vi "Open 4 Talon.vi"   [LabVIEW 2017]
uses:
  <vilib>/Rock Robotics/WPI/ThirdParty/Phoenix-LabVIEW/Motor Controller/Controls/CTRE_Phoenix_MotorControl_NeutralMode.ctl
  <vilib>/Rock Robotics/WPI/RobotDrive/WPI_RobotDriveOpen2MotorWithExistingMotors.vi
types:
  T1 = typedef "CTRE_Phoenix_MotorControl_NeutralMode.ctl" = enum8{"EEPROMSetting", "Override to Coast", "Override to Brake"}
  T2 = typedef "WPI_MotorControlDeviceRef.ctl" = cluster{"DeviceStatus":errorcluster, "Type":T3, "PWM":cluster{"PWM Channel":T4, "DeadBand":T5}, "CAN":cluster{"Device Number":u8, "SetOutput VI Ref":variant, "GetOutput VI Ref":variant, "Enable VI Ref":variant, "Disable VI Ref":variant, "Data":variant}, "Invert":bool, "DIO PWM":cluster{"PWM \"Enable\" Channel":T4, "DIOChannel":T6, "PWM Rate":dbl}}
  T3 = typedef "WPI_MotorControlType.ctl" = enum16{"PWM", "CAN", "DIO PWM"}
  T4 = typedef "FPGA_DIOPWMChannel.ctl" = enum8{"PWM 0", "PWM 1", "PWM 2", "PWM 3", "PWM 4", "PWM 5", "PWM 6", "PWM 7", "PWM 8", "PWM 9", "PWM MXP 0", "PWM MXP 1", "PWM MXP 2", "PWM MXP 3", "PWM MXP 4", "PWM MXP 5", "PWM MXP 6", "PWM MXP 7", "PWM MXP 8", "PWM MXP 9", "Invalid"}
  T5 = typedef "WPI_PWMDeadband.ctl" = cluster{"Name":string, "maxPositivePwm":i32, "minPositivePwm":i32, "centerPwm":i32, "maxNegativePwm":i32, "minNegativePwm":i32, "angularRange":u16}
  T6 = typedef "FPGA_DIOChannel.ctl" = enum8{"DIO 0", "DIO 1", "DIO 2", "DIO 3", "DIO 4", "DIO 5", "DIO 6", "DIO 7", "DIO 8", "DIO 9", "DIO MXP 0", "DIO MXP 1", "DIO MXP 2", "DIO MXP 3", "DIO MXP 4", "DIO MXP 5", "DIO MXP 6", "DIO MXP 7", "DIO MXP 8", "DIO MXP 9", "DIO MXP 10", "DIO MXP 11", "DIO MXP 12", "DIO MXP 13", "DIO MXP 14", "DIO MXP 15", "SPI Port CS1", "SPI Port CS2", "SPI Port CS3", "SPI Port MISO", "SPI Port MOSI", "Invalid"}
  T7 = typedef "WPI_RobotDriveDevRef.ctl" = cluster{"DevStatus":errorcluster, "Motors[]":T2[], "Square Inputs":bool, "Max Output":dbl}
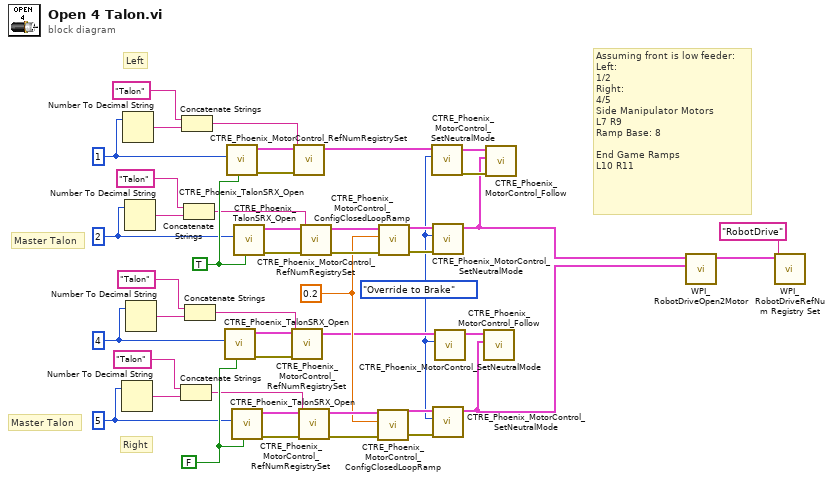
[diagram p0: block diagram]
diagram:
  w6 = CTRE_Phoenix_MotorControl_NeutralMode."Override to Brake" ("Motor Control Neutral Mode")
  w15 = 0.2 ("secondsFromNeutralToFull")
  w26 = FALSE ("Invert")
  w27 = TRUE ("Invert")
  w9 = u8 5 ("Device Number")
  w10 = u8 4 ("Device Number")
  w23 = u8 2 ("Device Number")
  w25 = u8 1 ("Device Number")
  # "Right"
  # "Left"
  # "Master Talon"
  # "Master Talon"
  # "Assuming front is low feeder:\nLeft:\n1/2\nRight:\n4/5\nSide Manipulator Motors\nL7 R9\nRamp Base: 8\n\nEnd Game Ramps\nL10 R11"
  n1 = Number To Decimal String(number=w9) -> (decimal integer string=w32:string)  [unwired: 1 in]
  n2 = Number To Decimal String(number=w25) -> (decimal integer string=w37:string)  [unwired: 1 in]
  n3 = Number To Decimal String(number=w23) -> (decimal integer string=w34:string)  [unwired: 1 in]
  n4 = Number To Decimal String(number=w10) -> (decimal integer string=w33:string)  [unwired: 1 in]
  n5 = Concatenate Strings("Talon", w32) -> (w20:string)
  n6 = Concatenate Strings("Talon", w37) -> (w24:string)
  n7 = Concatenate Strings("Talon", w34) -> (w22:string)
  n8 = Concatenate Strings("Talon", w33) -> (w21:string)
  n9 = call <vilib>:"CTRE_Phoenix_TalonSRX_Open.vi"("Invert"=w26, "Device Number"=w10) -> ("error out"=w42:errorcluster, "CAN Talon SRX Ref"=w45:T2)  [unwired: 8 in]
  n10 = call <vilib>:"CTRE_Phoenix_TalonSRX_Open.vi"("Invert"=w27, "Device Number"=w25) -> ("error out"=w41:errorcluster, "CAN Talon SRX Ref"=w38:T2)  [unwired: 8 in]
  n11 = call <vilib>:"CTRE_Phoenix_TalonSRX_Open.vi"("Invert"=w26, "Device Number"=w9) -> ("error out"=w43:errorcluster, "CAN Talon SRX Ref"=w44:T2)  [unwired: 8 in]
  n12 = call <vilib>:"CTRE_Phoenix_TalonSRX_Open.vi"("Invert"=w27, "Device Number"=w23) -> ("error out"=w40:errorcluster, "CAN Talon SRX Ref"=w39:T2)  [unwired: 8 in]
  n13 = call <vilib>:"CTRE_Phoenix_MotorControl_RefNumRegistrySet.vi"("error in (no error)"=w42, "refnum name"=w21, "PhoenixMotorControlDevRef"=w45) -> ("PhoenixMotorControlDevRef"=w7:T2)  [unwired: 7 in, 1 out]
  n14 = call <vilib>:"CTRE_Phoenix_MotorControl_RefNumRegistrySet.vi"("error in (no error)"=w41, "refnum name"=w24, "PhoenixMotorControlDevRef"=w38) -> ("PhoenixMotorControlDevRef"=w8:T2)  [unwired: 7 in, 1 out]
  n15 = call <vilib>:"CTRE_Phoenix_MotorControl_RefNumRegistrySet.vi"("error in (no error)"=w43, "refnum name"=w20, "PhoenixMotorControlDevRef"=w44) -> ("error out"=w19:errorcluster, "PhoenixMotorControlDevRef"=w18:T2)  [unwired: 7 in]
  n16 = call <vilib>:"CTRE_Phoenix_MotorControl_RefNumRegistrySet.vi"("error in (no error)"=w40, "refnum name"=w22, "PhoenixMotorControlDevRef"=w39) -> ("error out"=w16:errorcluster, "PhoenixMotorControlDevRef"=w17:T2)  [unwired: 7 in]
  n17 = call <vilib>:"CTRE_Phoenix_MotorControl_ConfigClosedLoopRamp.vi"("error in (no error)"=w19, "secondsFromNeutralToFull"=w15, "PhoenixMotorControlDevRef"=w18) -> ("error out"=w12:errorcluster, "PhoenixMotorControlDevRef"=w11:T2)  [unwired: 7 in]
  n18 = call <vilib>:"CTRE_Phoenix_MotorControl_ConfigClosedLoopRamp.vi"("error in (no error)"=w16, "secondsFromNeutralToFull"=w15, "PhoenixMotorControlDevRef"=w17) -> ("error out"=w13:errorcluster, "PhoenixMotorControlDevRef"=w14:T2)  [unwired: 7 in]
  n19 = call <vilib>:"CTRE_Phoenix_MotorControl_SetNeutralMode.vi"("Motor Control Neutral Mode"=w6, "PhoenixMotorControlDevRef"=w8) -> ("error out"=w4:errorcluster, "PhoenixMotorControlDevRef"=w5:T2)  [unwired: 8 in]
  n20 = call <vilib>:"CTRE_Phoenix_MotorControl_SetNeutralMode.vi"("error in (no error)"=w13, "Motor Control Neutral Mode"=w6, "PhoenixMotorControlDevRef"=w14) -> ("PhoenixMotorControlDevRef"=w1:T2)  [unwired: 7 in, 1 out]
  n21 = call <vilib>:"CTRE_Phoenix_MotorControl_SetNeutralMode.vi"("error in (no error)"=w12, "Motor Control Neutral Mode"=w6, "PhoenixMotorControlDevRef"=w11) -> ("PhoenixMotorControlDevRef"=w2:T2)  [unwired: 7 in, 1 out]
  n22 = call <vilib>:"CTRE_Phoenix_MotorControl_SetNeutralMode.vi"("Motor Control Neutral Mode"=w6, "PhoenixMotorControlDevRef"=w7) -> ("PhoenixMotorControlDevRef"=w3:T2)  [unwired: 8 in, 1 out]
  n23 = call <vilib>:"CTRE_Phoenix_MotorControl_Follow.vi"("Master Controller to Follow"=w2, "PhoenixMotorControlDevRef"=w3) -> ()  [unwired: 8 in, 2 out]
  n24 = call <vilib>:"CTRE_Phoenix_MotorControl_Follow.vi"("error in (no error)"=w4, "Master Controller to Follow"=w1, "PhoenixMotorControlDevRef"=w5) -> ()  [unwired: 7 in, 2 out]
  n25 = call-poly <vilib>:"WPI_RobotDriveOpen2Motor.vi"("Right Motor Dev Ref"=w2, "Left Motor Dev Ref"=w1) -> ("RobotDriveDevRef"=w29:T7)  [unwired: 8 in, 1 out]
  n26 = call <vilib>:"WPI_RobotDriveRefNum Registry Set.vi"("refnum name"="RobotDrive", "RobotDriveDevRef"=w29) -> ()  [unwired: 8 in, 2 out]
